vi "SDO download (array).vi"(6 "Value":u8[](array[numeric]), 7 "Wait?":bool, 8 "error in":errorcluster, 9 "Multiplexor":T1 {"Sub-Index" format="%.0x"; "Index" format="%04x"}, 10 "Node ID":u8, 11 "CANopen in":refnum<class "CANopen.lvclass">) -> (0 "error out":errorcluster, 3 "CANopen out":refnum<class "CANopen.lvclass">)   [LabVIEW 2026, in "canopen_.lvlib" / "CANopen.lvclass"]
doc: "Writes a value in the open dictionary of a CANopen node."
uses:
  CANopen.lvclass
  CANopen.lvclass/CANopen.ctl
  FunctionCode.ctl
  CANopen Master.lvlib
  Multiplexor.ctl
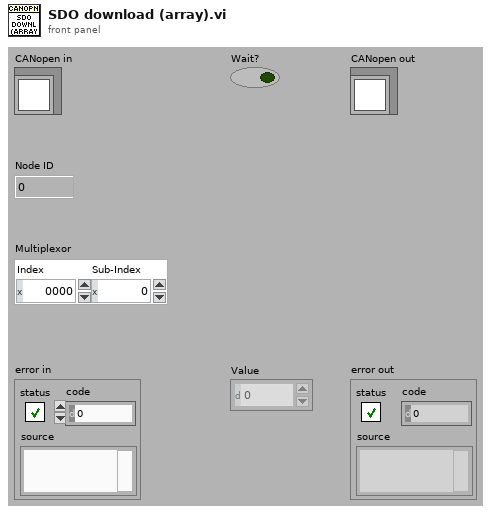
[diagram p1: front panel]
types:
  T1 = typedef "CANopen Master.lvlib/Multiplexor.ctl" = cluster{"Index":u16, "Sub-Index":i16}
  T2 = typedef "CANopen Master.lvlib/FunctionCode.ctl" = u16
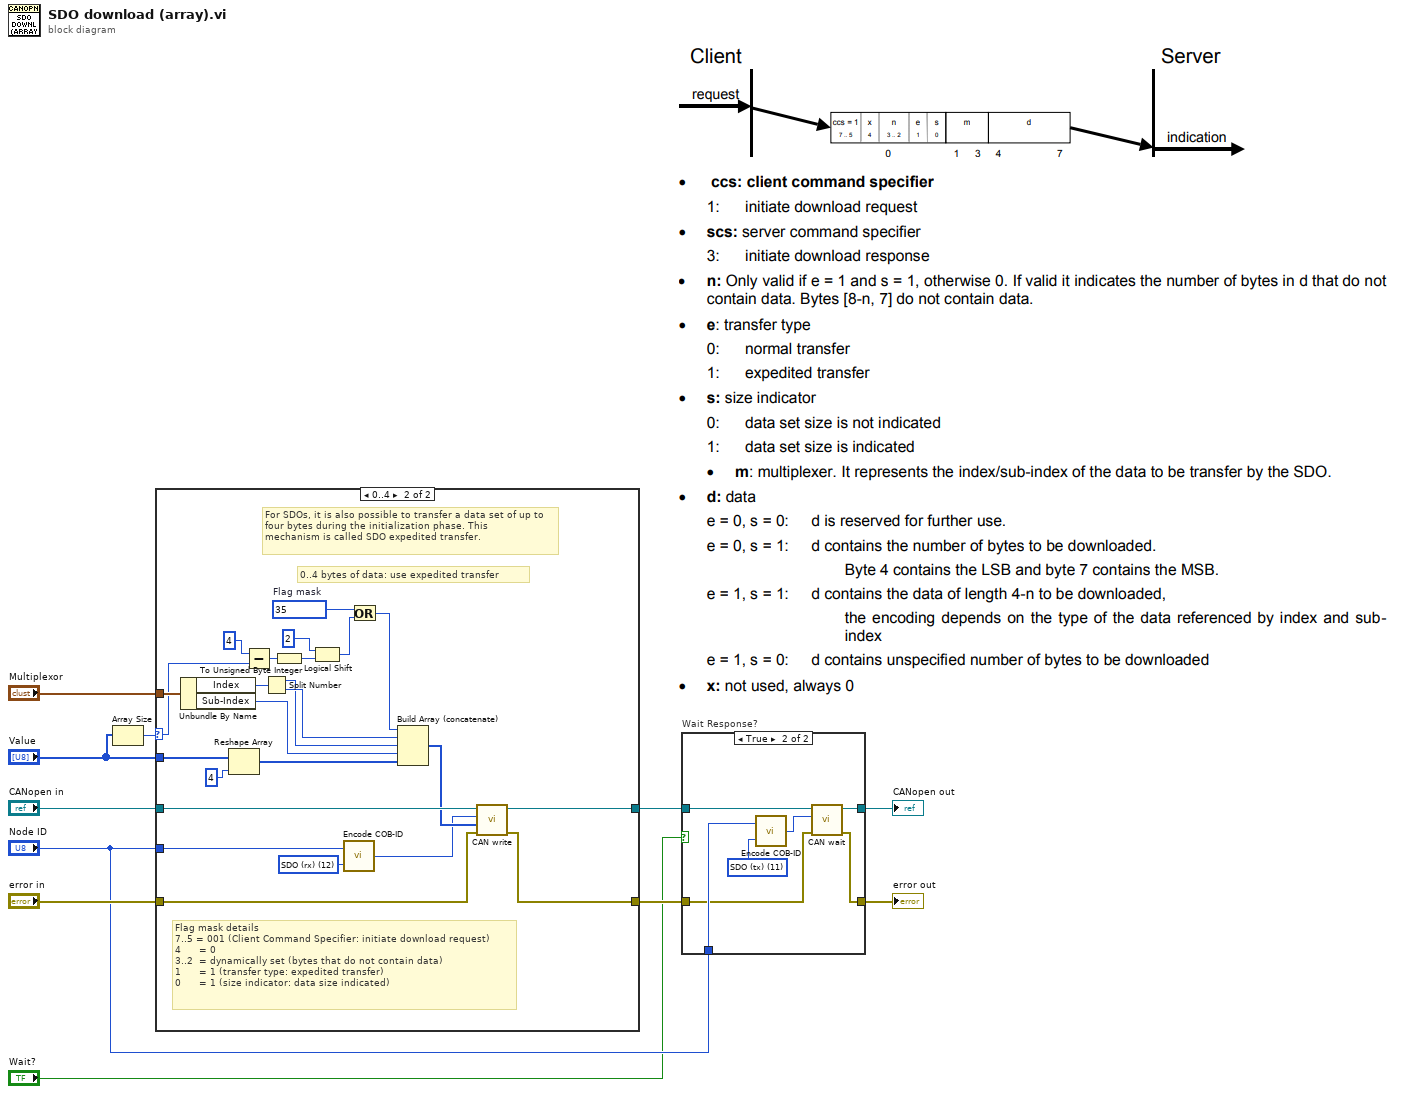
[diagram p0: block diagram]
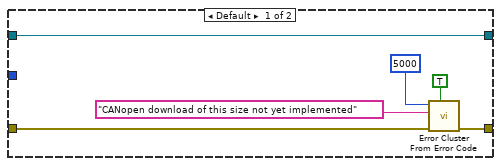
[diagram p2: hidden frame]
diagram:
  n1 = Array Size(array="Value") -> (size(s)=w10:i32)
  n2 = case shown="0..4" w10 {
    selector: w10 -> [_ w26]
    tunnel: "CANopen in" -> [w17 w41]
    tunnel: [w17 w40] -> w6
    tunnel: [w16 w39] -> w2
    tunnel: "Node ID" -> [_ w21]
    tunnel: "error in" -> [w13 w23]
    tunnel: "Value" -> [_ w30]
    tunnel: "Multiplexor" -> [_ w38]
    frame Default {
      n3 = call <vilib>:"Error Cluster From Error Code.vi"("show call chain? (False)"=TRUE, "error in (no error)"=w13, "error message (\"\")"="CANopen download of this size not yet implemented" ("source"), "error code (0)"=5000) -> ("error out"=w16:errorcluster)  [unwired: 5 in]
    }
    frame 0..4 {
      w19 = T2 12 items=["EMCY"=1, "PDO1 (tx)"=3, "PDO1 (rx)"=4, "PDO2 (tx)"=5, "PDO2 (rx)"=6, "PDO3 (tx)"=7, "PDO3 (rx)"=8, "PDO4 (tx)"=9, "PDO4 (rx)"=10, "SDO (tx)"=11, "SDO (rx)"=12, "NMT error control"=14] ("Function code")
      w31 = u8 35  # Flag mask
      # "For SDOs, it is also possible to transfer a data set of up to four bytes during the initialization phase. This \nmechanism is called SDO expedited transfer."
      # "Flag mask details\n7..5 = 001 (Client Command Specifier: initiate download request)\n4      = 0\n3..2  = dynamically set (bytes that do not contain data)\n1      = 1 (transfer type: expedited transfer)\n0      = 1 (size indicator: data size indicated)"
      # "0..4 bytes of data: use expedited transfer"
      n4 = Unbundle By Name(w38) -> ("Index"=w37:u16, "Sub-Index"=w34:i16)
      n5 = Reshape Array(w30, 4 ("y")) -> (w29:u8[])
      n6 = Subtract(x=4 ("y"), y=w26) -> (x-y=w27:i32)
      n7 = Split Number(x=w37) -> (hi(x)=w35:u8, lo(x)=w36:u8)
      n8 = To Unsigned Byte Integer(number=w27) -> (unsigned 8bit integer=w25:u8)
      n9 = Logical Shift(y=i8 2, x=w25) -> (x << y=w24:u8)
      n10 = call "Encode COB-ID.vi"("Function code"=w19, "Node-ID"=w21) -> ("COD-ID"=w20:u32)
      n11 = Or(x=w31, y=w24) -> (x .or. y?=w32:u8)
      n12 = Build Array (concatenate)(w32, w36, w35, w34, w29) -> (w22:i16[])
      n13 = call "CAN write.vi"("error in"=w23, "Data"=w22, "COB-ID"=w20, "CANopen in"=w41) -> ("error out"=w39:errorcluster, "CANopen out"=w40:refnum<class "CANopen.lvclass">)  [unwired: 6 in]
    }
  }
  n14 = case "Wait Response?" shown="True" "Wait?" {
    tunnel: w6 -> [w43 w49]
    tunnel: [w43 w48] -> w5
    tunnel: "Node ID" -> [_ w47]
    tunnel: [w42 w46] -> w3
    tunnel: w2 -> [w42 w45]
    frame False {
    }
    frame True {
      w50 = T2 11 items=["EMCY"=1, "PDO1 (tx)"=3, "PDO1 (rx)"=4, "PDO2 (tx)"=5, "PDO2 (rx)"=6, "PDO3 (tx)"=7, "PDO3 (rx)"=8, "PDO4 (tx)"=9, "PDO4 (rx)"=10, "SDO (tx)"=11, "SDO (rx)"=12, "NMT error control"=14] ("Function code")
      n15 = call "Encode COB-ID.vi"("Function code"=w50, "Node-ID"=w47) -> ("COD-ID"=w44:u32)
      n16 = call "CAN wait.vi"("error in"=w45, "COB-ID"=w44, "CANopen in"=w49) -> ("error out"=w46:errorcluster, "CANopen out"=w48:refnum<class "CANopen.lvclass">)  [unwired: 6 in, 1 out]
    }
  }
  "error out" <- w3
  "CANopen out" <- w5
